vi "ChooseSample.vi"(8 "In Sample Location":refnum<vi>, 11 "Sample locations of Interest":string[][](table)=[["X", "X", "X"], ["X", "X", ""], ["X", "X", "X"], ["X", "X", ""], ["X", "X", ""], ["X", "X", ""], ["X", "X", "X"], ["X", "X", ""], ["X", "", ""], ["X", "", ""], ["X", "", ""], ["", "", "X"], ["", "", "X"], ["", "", "X"], ["", "", ""]] caption="The spot: F5C in session; xrd_test") -> (1 "Selection Start":T1, 3 "Cancelled?":bool)   [LabVIEW 2010]
doc: "Use this template to create a dialog box with event handling."
uses:
  <vilib>/Utility/miscctls.llb/LVRowAndColumnTypeDef.ctl
panel:
  out "Column":i32
  out "Column Header Strings[]":string[](array[string])
  out "Valid Selection":bool
  in  "Cancel":bool
  in  "OK":bool
  # "Select a table cell with an X. The program will attempt to compute the transform from the spot\nselected below to the location in the coordinate system of the current session."
  # "Previous Sessions"
  # "Existing\nSpots"
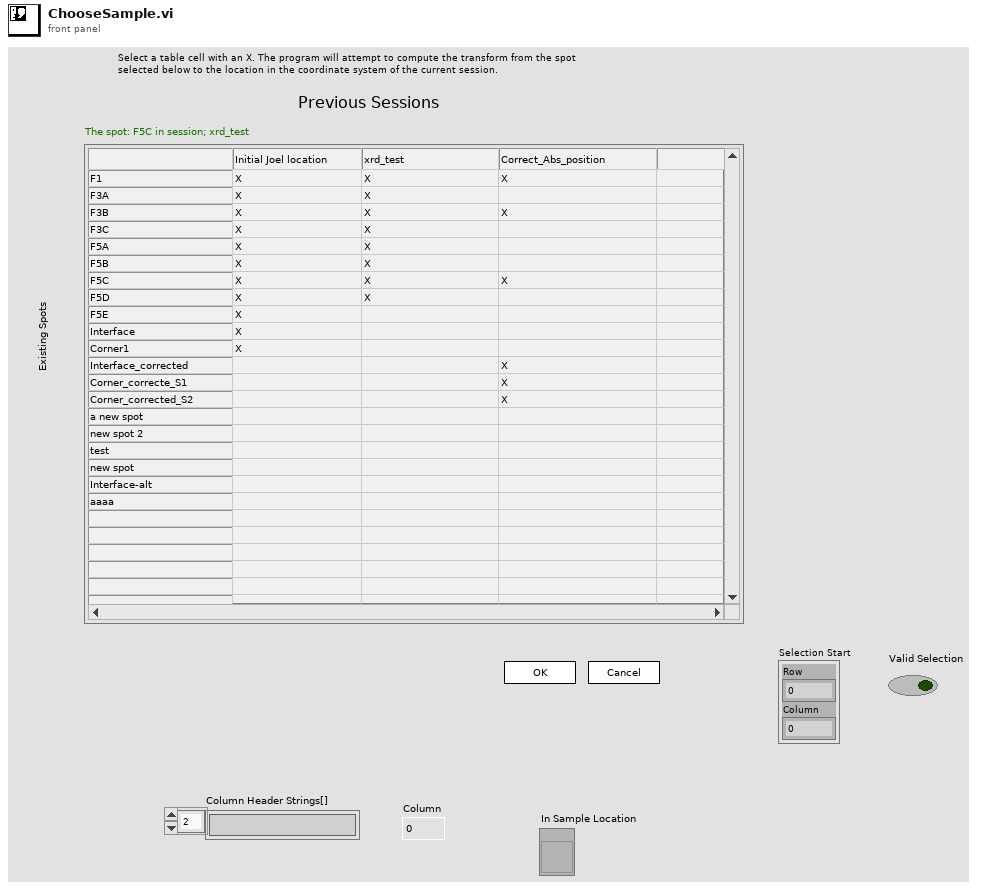
[diagram p1: front panel]
types:
  T1 = typedef "LVRowAndColumnTypeDef.ctl" = cluster{"Row":i32, "Column":i32}
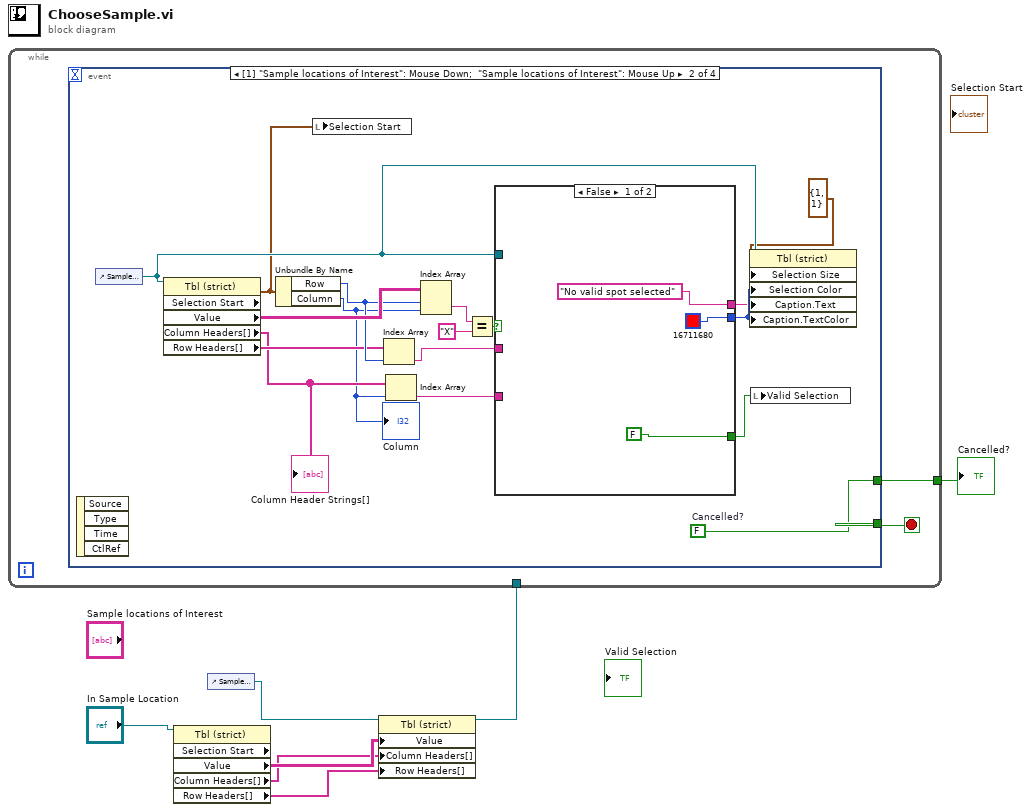
[diagram p0: block diagram]
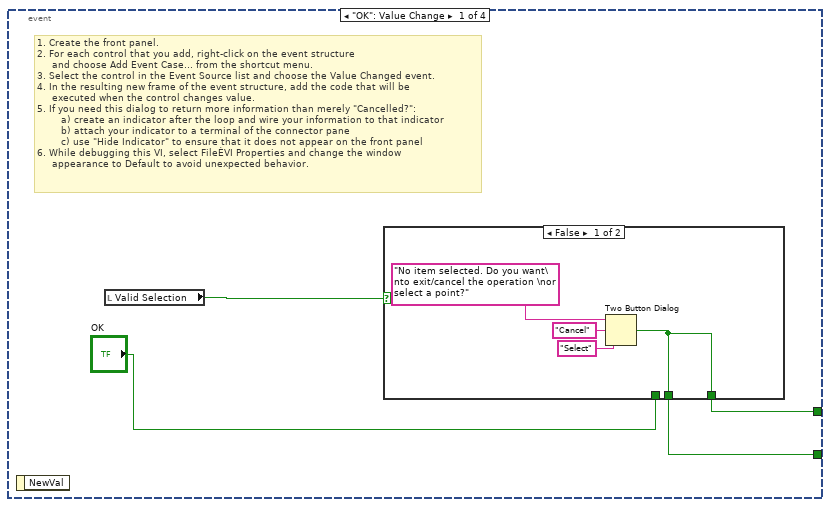
[diagram p2: hidden frame]
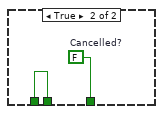
[diagram p3: hidden frame]
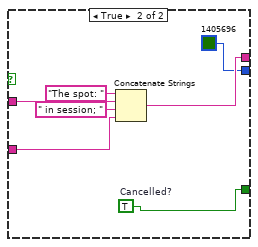
[diagram p4: hidden frame]
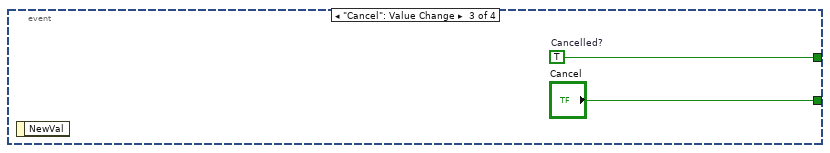
[diagram p5: hidden frame]
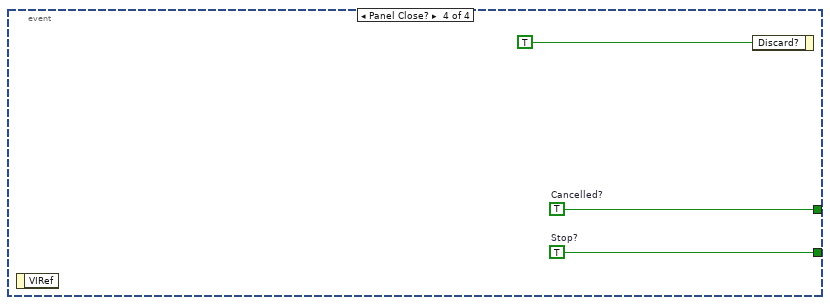
[diagram p6: hidden frame]
diagram:
  n1 = property class="Tbl (strict)" props=["Selection Start", "Value", "Column Headers[]", "Row Headers[]"](reference="In Sample Location") -> ("Value"=w4:string[][], "Column Headers[]"=w3:string[], "Row Headers[]"=w2:string[])  [unwired: 1 in, 3 out]
  n2 = control-ref of="Sample locations of Interest"() -> (w5:refnum<vi>)
  n3 = property class="Tbl (strict)"(reference=w5, "Value"=w4, "Column Headers[]"=w3, "Row Headers[]"=w2) -> (reference out=w1:refnum<vi>)  [unwired: 1 in, 1 out]
  n4 = while {
    tunnel: [w8] -> w7
    tunnel: w1 -> [_]
    stop <- w9 stop-if-true
    n5 = event shown="[1] \"Sample locations of Interest\": Mouse Down;  \"Sample locations of Interest\": Mouse Up" {
      selector: _ -> [_ _ _ _]
      dyn-events: _ -> [_ _ _ _]
      timeout: _ -> [_ _ _ _]
      tunnel: [w10 _ "Cancel" w50] -> w9
      tunnel: [w12 w20 w48 w49] -> w8
      event "OK": Value Change {
        # "1. Create the front panel.\n2. For each control that you add, right-click on the event structure \n     and choose Add Event Case... from the shortcut menu.\n3. Select the control in the Event Source list and choose the Value Changed event.\n4. In the resulting new frame of the event structure, add the code that will be \n     executed when the control changes value.\n5. If you need this dialog to return more information than merely \"Cancelled?\":\n        a) create an indicator after the loop and wire your information to that indicator\n        b) attach your indicator to a terminal of the connector pane\n        c) use \"Hide Indicator\" to ensure that it does not appear on the front panel\n6. While debugging this VI, select FileÈVI Properties and change the window \n     appearance to Default to avoid unexpected behavior."
        n6 = event-data() -> ()  [unwired: 1 in, 1 out]
        n7 = local read "Valid Selection"() -> (w13:bool)
        n8 = case shown="False" w13 {
          tunnel: [w14 w19] -> w12
          tunnel: "OK" -> [_ w18]
          tunnel: [w14 w18] -> w10
          frame False {
            n9 = Two Button Dialog(message="No item selected. Do you want\nto exit/cancel the operation \nor select a point?", 1:"Select" ("F button name (\"Cancel\")"), 2:"Cancel" ("T button name (\"OK\")")) -> (T button?=w14:bool)
          }
          frame True {
            w19 = FALSE  # Cancelled?
          }
        }
      }
      event "Sample locations of Interest": Mouse Down; "Sample locations of Interest": Mouse Up {
        w20 = FALSE  # Cancelled?
        n10 = event-data() -> ()  [unwired: 1 in, 4 out]
        n11 = control-ref of="Sample locations of Interest"() -> (w32:refnum<vi>)
        n12 = property class="Tbl (strict)"(reference=w32) -> ("Selection Start"=w22:T1, "Value"=w36:string[][], "Column Headers[]"=w28:string[], "Row Headers[]"=w29:string[])  [unwired: 1 in, 2 out]
        "Column Header Strings[]" <- w28
        n13 = Unbundle By Name(w22) -> ("Row"=w30:i32, "Column"=w27:i32)
        "Column" <- w27
        n14 = local write "Selection Start"(w22) -> ()
        n15 = Index Array(array=w29, index=w30) -> (element=w24:string)
        n16 = Index Array(array=w28, index=w27) -> (element=w23:string)
        n17 = Index Array(array=w36, index (row)=w30, index (col)=w27) -> (element=w35:string)
        n18 = Equal?(x=w35, y="X") -> (x = y?=w33:bool)
        n19 = case shown="False" w33 {
          tunnel: w32 -> [_ _]
          tunnel: [u32 16711680 ("Color") u32 1405696 ("Color")] -> w26
          tunnel: ["No valid spot selected" ("Label.Text") w42] -> w25
          tunnel: w24 -> [_ w46]
          tunnel: w23 -> [_ w45]
          tunnel: [FALSE ("Cancelled?") w40] -> w21
          frame False {
          }
          frame True {
            w40 = TRUE  # Cancelled?
            n20 = Concatenate Strings("The spot: " ("string"), w46, " in session; " ("string"), w45) -> (w42:string)
          }
        }
        n21 = property class="Tbl (strict)"(reference=w32, "Selection Size"=T1 {"Row"=1, "Column"=1}, "Selection Color"=w26, "Caption.Text"=w25, "Caption.TextColor"=w26) -> ()  [unwired: 1 in, 2 out]
        n22 = local write "Valid Selection"(w21) -> ()
      }
      event "Cancel": Value Change {
        w48 = TRUE  # Cancelled?
        n23 = event-data() -> ()  [unwired: 1 in, 1 out]
      }
      event Panel Close? {
        w49 = TRUE  # Cancelled?
        w50 = TRUE  # Stop?
        n24 = event-data() -> ()  [unwired: 1 in, 1 out]
        n25 = event-data("Discard?"=TRUE) -> ()  [unwired: 1 in, 1 out]
      }
    }
  }
  "Cancelled?" <- w7
